vi "S2C_PCIe1762H_Proc_DigitalWrite.vi"(8 "Error In":errorcluster, 11 "FootSwitch":string) -> (0 "Error Out":errorcluster, 3 "Result":string)   [LabVIEW 2024]
uses:
  TypeDefs/S2C_PCIe1762H_Type_FootSwitch.ctl
  S2C_PCIe1762H_Proc_Globals.vi
  <userlib>/DAQNavi Polymorphic VI/create/DAQNavi Create Channel(DO-Digital Output).vi
  <userlib>/DAQNavi Polymorphic VI/write/DAQNavi Write (Digital U8 1Chan 1Samp).vi
  <userlib>/DAQNavi Polymorphic VI/read/DAQNavi Read (Digital U8 1Chan 1Samp).vi
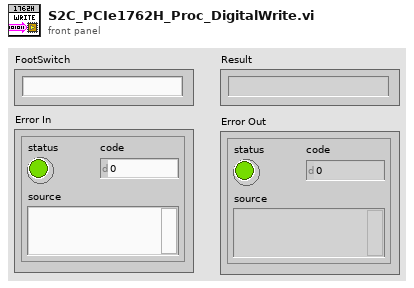
[diagram p1: front panel]
types:
  T1 = typedef "S2C_PCIe1762H_Type_FootSwitch.ctl" = u16
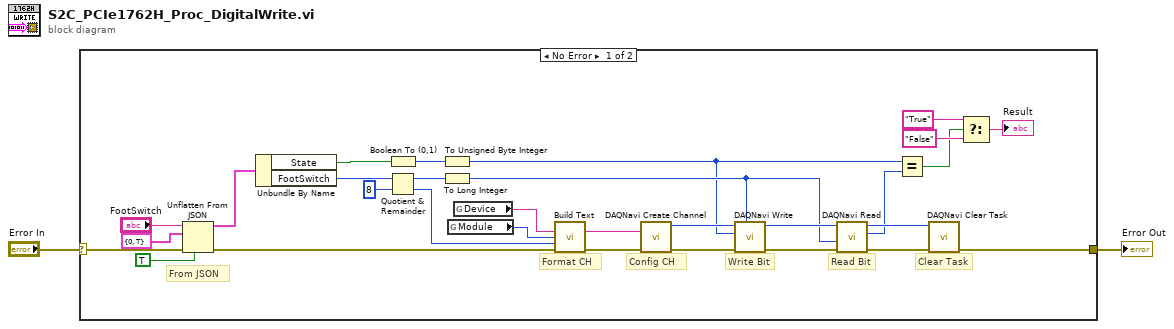
[diagram p0: block diagram]
diagram:
  n1 = case shown="No Error" "Error In" {
    selector: "Error In" -> [w6 w33]
    tunnel: [w5 w33] -> w1
    frame No Error {
      # "Clear Task"
      # "Read Bit"
      # "Write Bit"
      # "Format CH"
      # "Config CH"
      # "From JSON"
      n2 = Unflatten From JSON(JSON string="FootSwitch", type and defaults=cluster{"FootSwitch":T1, "State":bool} {"FootSwitch"=0, "State"=TRUE}, default null elements? (F)=TRUE, error in (no error)=w6) -> (value=w29:cluster{"FootSwitch":T1, "State":bool}, error out=w28:errorcluster)  [unwired: 3 in]
      n3 = Unbundle By Name(w29) -> ("State"=w20:bool, "FootSwitch"=w27:T1)
      n4 = Boolean To (0,1)(Boolean=w20) -> (0, 1=w19:i16)
      n5 = Quotient & Remainder(x=w27, y=u16 8) -> (x-y*floor(x/y)=w16:T1, floor(x/y)=w21:T1)
      n6 = To Unsigned Byte Integer(number=w19) -> (unsigned 8bit integer=w11:u8)
      n7 = To Long Integer(number=w16) -> (32bit integer=w15:i32)
      n8 = global read "S2C_PCIe1762H_Proc_Globals.vi" "Module"() -> (w4:i32)
      n9 = global read "S2C_PCIe1762H_Proc_Globals.vi" "Device"() -> (w3:string)
      n10 = call "Build Text"("Device"=w3, "Module"=w4, "Port"=w21, "error in (no error)"=w28) -> ("Result"=w24:string, "error out"=w25:errorcluster)  [unwired: 10 in]
      n11 = call-poly <userlib>:"DAQNavi Create Channel.vi"("physical channels"=w24, "error in (no error)"=w25) -> ("task out"=w22:i32, "error out"=w23:errorcluster)  [unwired: 3 in, 9 out]
      n12 = call-poly <userlib>:"DAQNavi Write.vi"("portBit"=w15, "error in (no error)"=w23, "data"=w11, "task in"=w22) -> ("error out"=w18:errorcluster, "task out"=w17:i32)  [unwired: 1 in, 5 out]
      n13 = call-poly <userlib>:"DAQNavi Read.vi"("error in (no error)"=w18, "portBit"=w15, "task in"=w17) -> ("error out"=w14:errorcluster, "data"=w12:u8, "task out"=w13:i32)  [unwired: 1 in, 5 out]
      n14 = Equal?(x=w11, y=w12) -> (x = y?=w8:bool)
      n15 = call <userlib>:"DAQNavi Clear Task.vi"("error in (no error)"=w14, "task in"=w13) -> ("error out"=w5:errorcluster)  [unwired: 1 out]
      n16 = Select(t="True", s=w8, f="False") -> (s? t:f=→"Result":string)
    }
    frame Error {
    }
  }
  "Error Out" <- w1
